vi "Wake Up Time Out Event Case--constant.vi"() -> (3 "Wake up TimeOut Event Case":i32)   [LabVIEW 2018, in "Timer Module.lvlib"]
uses:
  Timer Module.lvlib
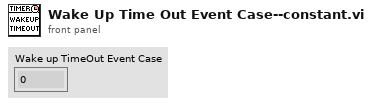
[diagram p1: front panel]
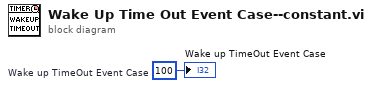
[diagram p0: block diagram]
diagram:
  w1 = 100  # Wake up TimeOut Event Case
  "Wake up TimeOut Event Case" <- w1
